vi "2-2-4.vi"() -> ()   [LabVIEW 2020]
panel:
  out "appended array 5":dbl[][](array[numeric])
  out "appended array 4":dbl[](array[numeric])
  out "appended array 2":dbl[](array[numeric])
  out "appended array 3":dbl[](array[numeric])
  out "appended array":dbl[](array[numeric])
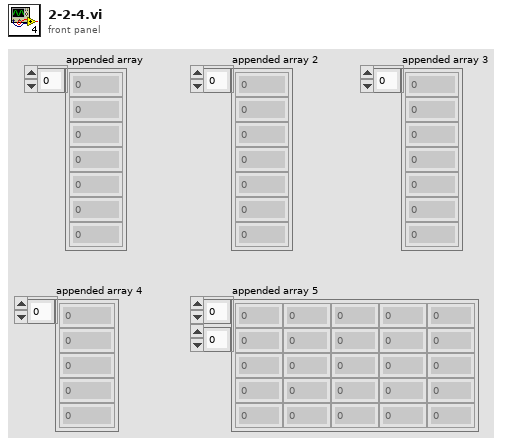
[diagram p1: front panel]
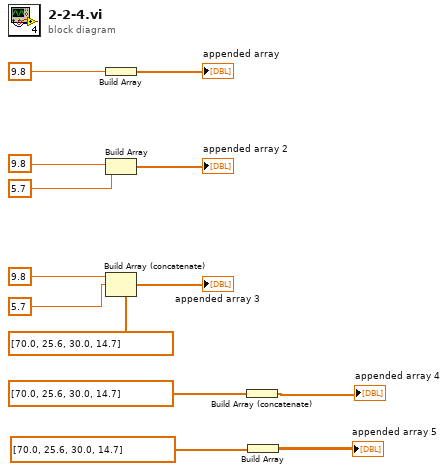
[diagram p0: block diagram]
diagram:
  n1 = Build Array(9.8 ("element")) -> (→"appended array":dbl[])
  n2 = Build Array(9.8 ("element 5"), 5.7 ("element 6")) -> (→"appended array 2":dbl[])
  n3 = Build Array (concatenate)(9.8 ("element 2"), 5.7 ("element 3"), dbl[] [70.0, 25.6, 30.0, 14.7]) -> (→"appended array 3":dbl[])
  n4 = Build Array (concatenate)(dbl[] [70.0, 25.6, 30.0, 14.7]) -> (→"appended array 4":dbl[])
  n5 = Build Array(dbl[] [70.0, 25.6, 30.0, 14.7]) -> (→"appended array 5":dbl[][])
